vi "Unknown State Error.vi"(8 "error in (no error)":errorcluster, 11 "state":string) -> (0 "error out":errorcluster)   [LabVIEW 2019, in "Routing and Faulting Scripting.lvlib"]
uses:
  Routing and Faulting Scripting.lvlib
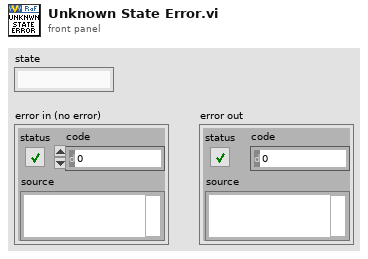
[diagram p1: front panel]
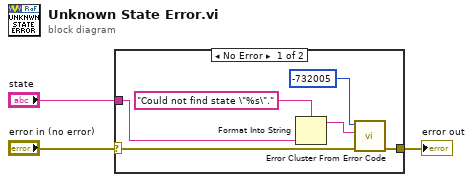
[diagram p0: block diagram]
diagram:
  n1 = case shown="No Error" "error in (no error)" {
    selector: "error in (no error)" -> [w5 w10]
    tunnel: "state" -> [w7 _]
    tunnel: [w6 w10] -> w2
    frame No Error {
      n2 = Format Into String(format string="Could not find state \"%s\".", w7) -> (resulting string=w9:string)  [unwired: 2 in, 1 out]
      n3 = call <vilib>:"Error Cluster From Error Code.vi"("error in (no error)"=w5, "error message (\"\")"=w9, "error code (0)"=-732005) -> ("error out"=w6:errorcluster)  [unwired: 6 in]
    }
    frame Error {
    }
  }
  "error out" <- w2
